vi "Insight_Calibrate_Sweep.vi"(8 "error in (no error)":errorcluster, 9 "Mode (Read / Write)":enum8{"Write", "Read"}(ring), 11 "telnet connection":T1) -> (0 "error out":errorcluster, 1 "response data":string, 3 "telnet  connection out":T1)   [LabVIEW 2014]
doc: "Insight Photonic Solutions\n\nThis VI commands the laser to perform a calibration of the laser sweep.\n\nver 1.0 - original release\nver 1.1 - added response data buffer as an output\nver 3.2 - added query option, part of Atlas 3.2 in the laser software, which returns the quality of the sweep calibration after calibration."
uses:
  Telnet Session.ctl
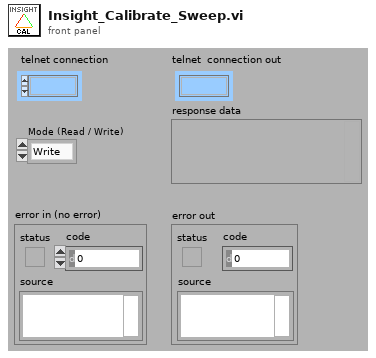
[diagram p1: front panel]
types:
  T1 = typedef "Telnet Session.ctl" = refnum<k1>
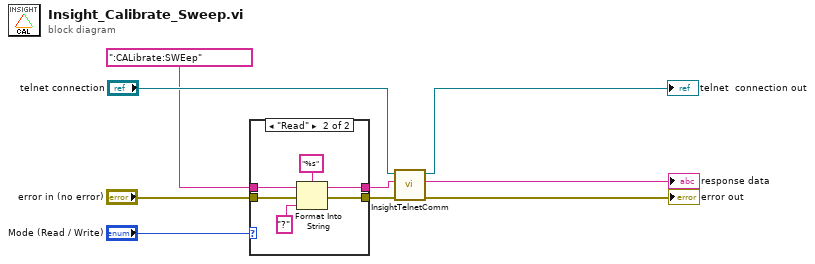
[diagram p0: block diagram]
diagram:
  n1 = case shown="\"Read\"" "Mode (Read / Write)" {
    tunnel: [w10 w13] -> w2
    tunnel: "error in (no error)" -> [w10 w12]
    tunnel: ":CALibrate:SWEep" ("String") -> [w11 w15]
    tunnel: [w11 w14] -> w1
    frame "Write", Default {
    }
    frame "Read" {
      n2 = Format Into String(format string="%s", initial string=w15, error in=w12, "?" ("input 1")) -> (resulting string=w14:string, error out=w13:errorcluster)
    }
  }
  n3 = call "InsightTelnetComm.vi"("error in"=w2, "write buffer (\"\")"=w1, "telnet connection"="telnet connection") -> ("error out"=→"error out":errorcluster, "response data"=→"response data":string, "telnet  connection out"=→"telnet  connection out":T1)  [unwired: 4 in]
